vi "McP Serial INIT v0.49.vi"(2 "error in (no error)":errorcluster) -> (0 "Error out":errorcluster, 1 "Serial PortNumber":i32)   [LabVIEW 2019]
doc: "This Vi initialize the McPherson spectrometer and the serial port connected to it. The port number is a global variable, and do not need to be wired."
uses:
  Globals and TypeDefs/Global Varibal Control.vi
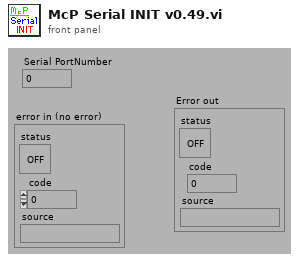
[diagram p1: front panel]
types:
  T1 = enum16{"no parity", "odd parity", "even parity", "mark parity", "space parity"}
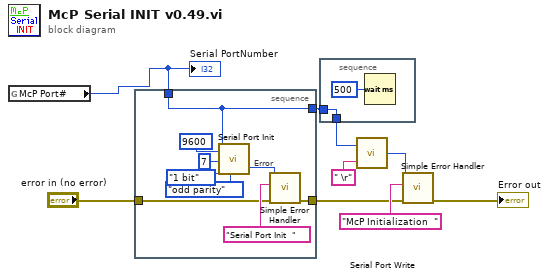
[diagram p0: block diagram]
diagram:
  n1 = global read "Global Varibal Control.vi" "McP Port#"() -> (w1:i32)
  "Serial PortNumber" <- w1
  n2 = stacked-sequence {
    tunnel: "error in (no error)" -> [w12]
    tunnel: w1 -> [w11]
    tunnel: [w11] -> w4
    tunnel: [w10] -> w7
    frame #0 {
      # "Error"
      n3 = call <vilib>:"Serial Port Init.vi"("parity"=T1."odd parity", "stop bits"=enum16{"1 bit", "1.5 bits", "2 bits"}."1 bit", "data bits"=u16 7, "baud rate"=u16 9600, "port number"=w11) -> ("error code"=w16:i32)  [unwired: 2 in]
      n4 = call <vilib>:"Simple Error Handler.vi"("error code (no error:0)"=w16, "error source (\" \")"="Serial Port Init  ", "error in (no error)"=w12) -> ("error out"=w10:errorcluster)  [unwired: 2 in, 4 out]
    }
  }
  n5 = stacked-sequence {
    tunnel: [w19] -> w2
    tunnel: w4 -> [w19]
    frame #0 {
      n6 = Wait (ms)(milliseconds to wait=u32 500) -> ()  [unwired: 1 out]
    }
  }
  n7 = call <vilib>:"Serial Port Write.vi"("string to write"=" \r", "port number"=w2) -> ("error code"=w3:i32)
  n8 = call <vilib>:"Simple Error Handler.vi"("error code (no error:0)"=w3, "error source (\" \")"="McP Initialization  ", "error in (no error)"=w7) -> ("error out"=→"Error out":errorcluster)  [unwired: 2 in, 4 out]
